vi "Set Standard Event Register.vi"(0 "VISA resource name":refnum<visa-resource-name>, 7 "Standard Event Register":u8, 11 "error in (no error)":errorcluster) -> (4 "VISA resource name out":refnum<visa-resource-name>, 15 "error out":errorcluster)   [LabVIEW 2016, in "eec EST 300.lvlib"]
doc: "*ESE <value>\nStandard Event enable register controls which bits will be logically ORed together to generate the Event Summary bit 5 (ESB) within the Status Byte."
uses:
  <instrlib>/eec EST 300/eec EST 300.lvlib
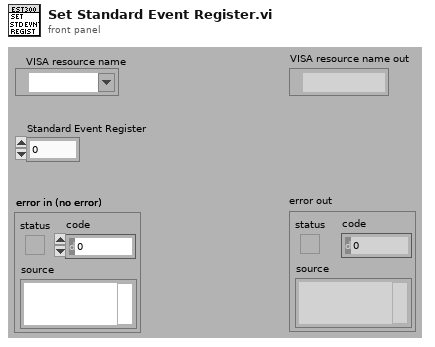
[diagram p1: front panel]
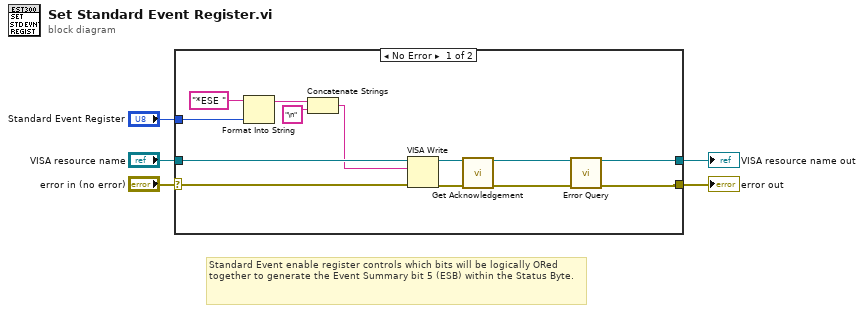
[diagram p0: block diagram]
diagram:
  # "Standard Event enable register controls which bits will be logically ORed together to generate the Event Summary bit 5 (ESB) within the Status Byte."
  n1 = case shown="No Error" "error in (no error)" {
    selector: "error in (no error)" -> [w17 w20]
    tunnel: [w10 w20] -> w4
    tunnel: [w11 w19] -> w2
    tunnel: "VISA resource name" -> [w18 w19]
    tunnel: "Standard Event Register" -> [w15 _]
    frame No Error {
      n2 = Format Into String(initial string="*ESE " ("Command to Send"), w15) -> (resulting string=w14:string)  [unwired: 2 in, 1 out]
      n3 = Concatenate Strings(w14, "\n" ("string")) -> (w13:string)
      n4 = VISA Write(VISA resource name=w18, write buffer=w13, error in (no error)=w17) -> (VISA resource name out=w7:refnum<visa-resource-name>, error out=w6:errorcluster)  [unwired: 1 out]
      n5 = call <instrlib>:"Get Acknowledgement.vi"("VISA resource name"=w7, "error in (no error)"=w6) -> ("VISA resource name out"=w8:refnum<visa-resource-name>, "error out"=w9:errorcluster)  [unwired: 12 in]
      n6 = call <instrlib>:"Error Query.vi"("VISA resource name"=w8, "error in (no error)"=w9) -> ("VISA resource name out"=w11:refnum<visa-resource-name>, "error out"=w10:errorcluster)  [unwired: 10 in, 2 out]
    }
    frame Error {
    }
  }
  "error out" <- w4
  "VISA resource name out" <- w2
